vi "NI_FPGA_PPG.set pattern time value.vi"(0 "i ref in":refnum<vi>, 1 "memory_addr":i32, 2 "time [us]":dbl, 3 "ms timeout (10000)":i32=10000, 5 "error in (no error)":errorcluster) -> (14 "i ref out":refnum<vi>, 17 "timed out":bool, 19 "error out":errorcluster)   [LabVIEW 2014, in "NI_FPGA_PPG.lvlib"]
doc: "Sets new time value for specified time pattern. The memory address must refer to a \"$time$ command.\n\nLicense Agreement for this software:\n\nCopyright (C) 2009\nFalk Ziegler\nInstitut für Physik\nErnst-Moritz-Arndt Universität\nFelix-Hausdorff-Str. 6\n17487 Greifswald\n\nContact: Falk Ziegler, ziegler@physik.uni-greifswald.de\n\nThis program is free software: you can redistribute it and/or modify it under the terms of the GNU General Public License as published by the Free Software Foundation, either version 3 of the License, or (at your option) any later version.\n\nThis program is distributed in the hope that it will be useful, but WITHOUT ANY WARRANTY; without even the implied warranty of MERCHANTABILITY or FITNESS FOR A PARTICULAR PURPOSE. See the GNU General Public License for more details.\n\nYou should have received a copy of the GNU General Public License along with this program. If not, see <http://www.gnu.org/licenses/>.\n\nFor all questions and ideas contact: ziegler@physik.uni-greifswald.de or d.beck@gsi.de\nLast update: 01-Sep-2009"
uses:
  NI_FPGA_PPG.lvlib
  CSCore/CSSystem/CoreDefs/CoreDefs.error_type.ctl
  CSCore/CSSystem/CoreDefs/CoreDefs.error_severity.ctl
  CSCore/CSApplicationBaseClasses/DeviceBase/DeviceBase.lvlib
  CSinstr.lib/NI_FPGA_PPG/host/instrumentDriver/NI-FPGA_PPG_Driver.lvlib
  CSCore/CSSystem/CoreLib/CoreLib.lvlib
  CSlibraries/UtilityLib/UtilityLib.lvlib
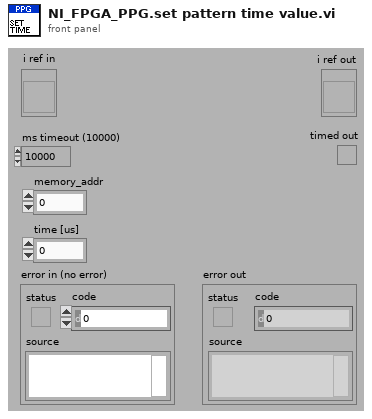
[diagram p1: front panel]
types:
  T1 = typedef "CoreDefs.error_severity.ctl" = enum16{"undefined", "information", "warning", "error", "fatal"}
  T2 = typedef "CoreDefs.error_type.ctl" = enum16{"no error", "can't load process", "can't unload process", "process does not exist", "can't install process", "can't remove process", "unknown function", "time out", "can't execute function", "duplicate queue name", "super not found", "caller queue invalid", "can't ping process", "unknown error", "VISA Error", "VISA timeout", "GPIB timeout", "GPIB error", "communication error", "data type mismatch", "can't read data from OPC server", "can't write data to OPC server", "OET error", "function not implemented", "process already exists", "invalid Shared Variable name", "error writing Shared Variable", "error reading Shared Variable", "invalid client name", "corrupt database", "unknown class", "call not authorized", "parameter out of range", "OET timeout: can't get data to modify", "invalid queue name", "requested operation incompatible with current state", "event undefined", "event disabled", "state undefined", "caller is not a friend", "EventBuilder: bad eventID", "EventBuilder: no DAQ devices", "a thread must not stop itself", "UNUSED ELEMENT4", "DiscArchiver: eventData incomplete", "DiscArchiver: eventData does not belong to run", "DiscArchiver: can't open file", "DiscArchiver: can't write to file", "DiscArchiver: available disc space low", "can't acquire semaphore", "error reading data from database", "notifier object is not existing", "can't register process", "can't unregister process", "illegal event type", "object disabled", "object already exists", "can't change state", "Instrument not found", "no connection to remote node", "invalid reference", "N/A", "UNUSED ELEMENT 1", "element not found", "illegal TCP/IP connection detected", "object does not exist", "invalid access ID", "unknown CS system", "invalid privilige", "unsupported data type", "unsupported server type", "IO server already exists", "Shared Variable already exists"}
  T3 = typedef "NI_FPGA_PPG.lvlib/NI_FPGA_PPG.i attribute.ctl" = cluster{"dim_service_id":cluster{"dim_actual_device_status":i32, "dim_event_data":i32, "dim_cmd_data":i32, "dim_cmd_data _description":i32, "dim_channel_description":i32}, "VISA":refnum<visa-resource-name>, "actual_device_status":i32, "event_data_id":i32, "pdc_enabled":bool, "pdc_timestamp":u32, "cmd_data_string":string, "cmd_data_size":i32, "cmd_data_description_string":string, "cmd_data_description_size":i32, "channel_description_string":string, "channel_description_size":i32}
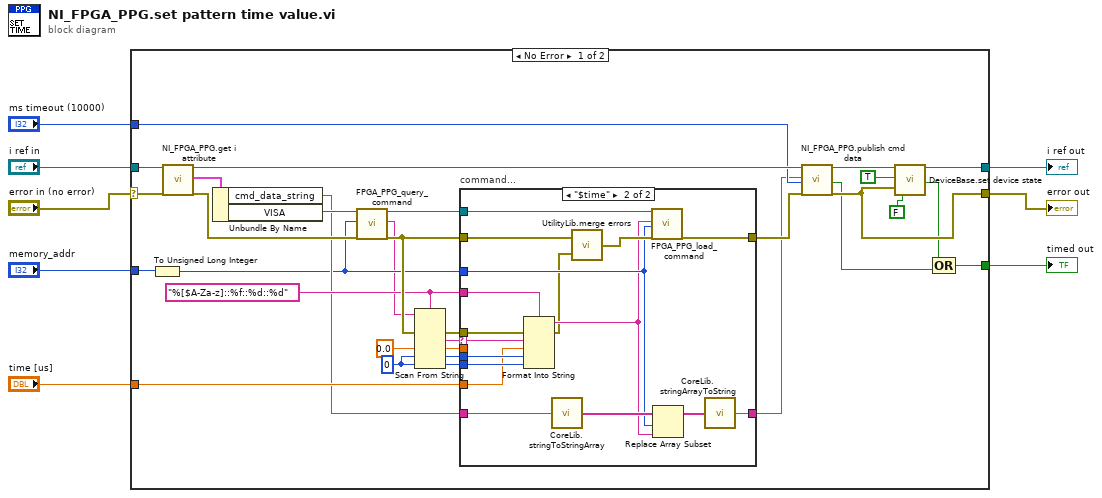
[diagram p0: block diagram]
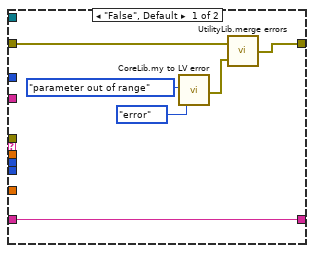
[diagram p2: hidden frame]
diagram:
  n1 = case shown="No Error" "error in (no error)" {
    selector: "error in (no error)" -> [w38 w64]
    tunnel: "i ref in" -> [w39 w65]
    tunnel: [w34 w65] -> w6
    tunnel: [w18 w64] -> w5
    tunnel: "ms timeout (10000)" -> [w19 _]
    tunnel: "memory_addr" -> [w33 _]
    tunnel: "time [us]" -> [w22 _]
    tunnel: [w14 _] -> w1
    frame No Error {
      w30 = u32 0
      w23 = "%[$A-Za-z]::%f::%d::%d" ("format string")
      n2 = To Unsigned Long Integer(number=w33) -> (unsigned 32bit integer=w12:u32)
      n3 = call "NI_FPGA_PPG.get i attribute.vi"("i ref in"=w39, "error in (no error)"=w38) -> ("i ref out"=w20:refnum<vi>, "i attribute"=w35:T3, "error out"=w31:errorcluster)  [unwired: 15 in]
      n4 = Unbundle By Name(w35) -> ("cmd_data_string"=w13:string, "VISA"=w32:refnum<visa-resource-name>)
      n5 = call "FPGA_PPG_query_command.vi"("resource_in"=w32, "mem_addr"=w12, "error in (no error)"=w31) -> ("resource_out"=w26:refnum<visa-resource-name>, "command"=w11:string, "error out"=w40:errorcluster)  [unwired: 14 in]
      n6 = Scan From String(format string=w23, input string=w11, error in=w40, default 2=0.0 ("default value 2"), default 3=w30, default 4=w30) -> (error out=w25:errorcluster, output 1=w24:string, output 2=w29:dbl, output 3=w28:u32, output 4=w27:u32)  [unwired: 2 in, 2 out]
      n7 = case "command..." shown="\"$time\"" w24 {
        selector: w24 -> [_ w47]
        tunnel: w12 -> [_ w51]
        tunnel: w29 -> [_ _]
        tunnel: w28 -> [_ w60]
        tunnel: w27 -> [_ w59]
        tunnel: w22 -> [_ w57]
        tunnel: w26 -> [_ w63]
        tunnel: w40 -> [w45 w49]
        tunnel: [w41 w62] -> w10
        tunnel: w25 -> [_ w61]
        tunnel: w23 -> [_ w58]
        tunnel: w13 -> [w46 w55]
        tunnel: [w46 w52] -> w9
        frame "False", Default {
          n8 = call "CoreLib.my to LV error.vi"("ErrorTypes"=CoreDefs.error_type."parameter out of range", "severityLevel"=CoreDefs.error_severity."error") -> ("myErrorCluster"=w44:errorcluster)  [unwired: 16 in, 1 out]
          n9 = call "UtilityLib.merge errors.vi"("error2 (no error)"=w44, "error1 (no error)"=w45) -> ("error out"=w41:errorcluster)
        }
        frame "$time" {
          n10 = Format Into String(format string=w58, error in=w61, w47, w57, w60, w59) -> (resulting string=w50:string, error out=w48:errorcluster)  [unwired: 1 in]
          n11 = call "CoreLib.stringToStringArray.vi"("String"=w55) -> ("Array"=w54:string[])
          n12 = call "UtilityLib.merge errors.vi"("error2 (no error)"=w48, "error1 (no error)"=w49) -> ("error out"=w56:errorcluster)
          n13 = call "FPGA_PPG_load_command.vi"("resource_in"=w63, "command"=w50, "mem_addr"=w51, "error in (no error)"=w56) -> ("error out"=w62:errorcluster)  [unwired: 14 in, 1 out]
          n14 = Replace Array Subset(array=w54, new element=w50, index=w51) -> (w53:string[])
          n15 = call "CoreLib.stringArrayToString.vi"("Array"=w53) -> ("String"=w52:string)
        }
      }
      n16 = call "NI_FPGA_PPG.publish cmd data.vi"("i ref in"=w20, "cmd_data_string"=w9, "ms timeout (10000)"=w19, "error in (no error)"=w10) -> ("i ref out"=w17:refnum<vi>, "timed out"=w15:bool, "error out"=w18:errorcluster)  [unwired: 13 in]
      n17 = call "DeviceBase.set device state.vi"("i ref in"=w17, "implicit"=TRUE, "device error"=w18, "mayResetError (FALSE)"=FALSE) -> ("i ref out"=w34:refnum<vi>, "timed out"=w16:bool)  [unwired: 13 in, 1 out]
      n18 = Compound Arithmetic op=OR(w16, w15) -> (w14:bool)
    }
    frame Error {
    }
  }
  "error out" <- w5
  "i ref out" <- w6
  "timed out" <- w1
